vi "loadCTTAT.vi"() -> ()   [LabVIEW 2012]
uses:
  <vilib>/addons/database/Connection.llb/DB Tools Open Connec (Path).vi
  <vilib>/addons/database/Connection.llb/Conn Execute.vi
  <vilib>/addons/database/Recordset.llb/Rec Destroy - Connection.vi
  <vilib>/addons/database/Recordset.llb/Rec Fetch Recordset Data (R).vi
  <vilib>/addons/database/_DB Variant To Data/Database Variant To Data.xnode
  <vilib>/addons/database/NI_Database_API.lvlib
panel:
  out "date/time string":string
  out "recordset data":variant[][](array[variant])
  out "concatenated string":string
  out "error out":errorcluster
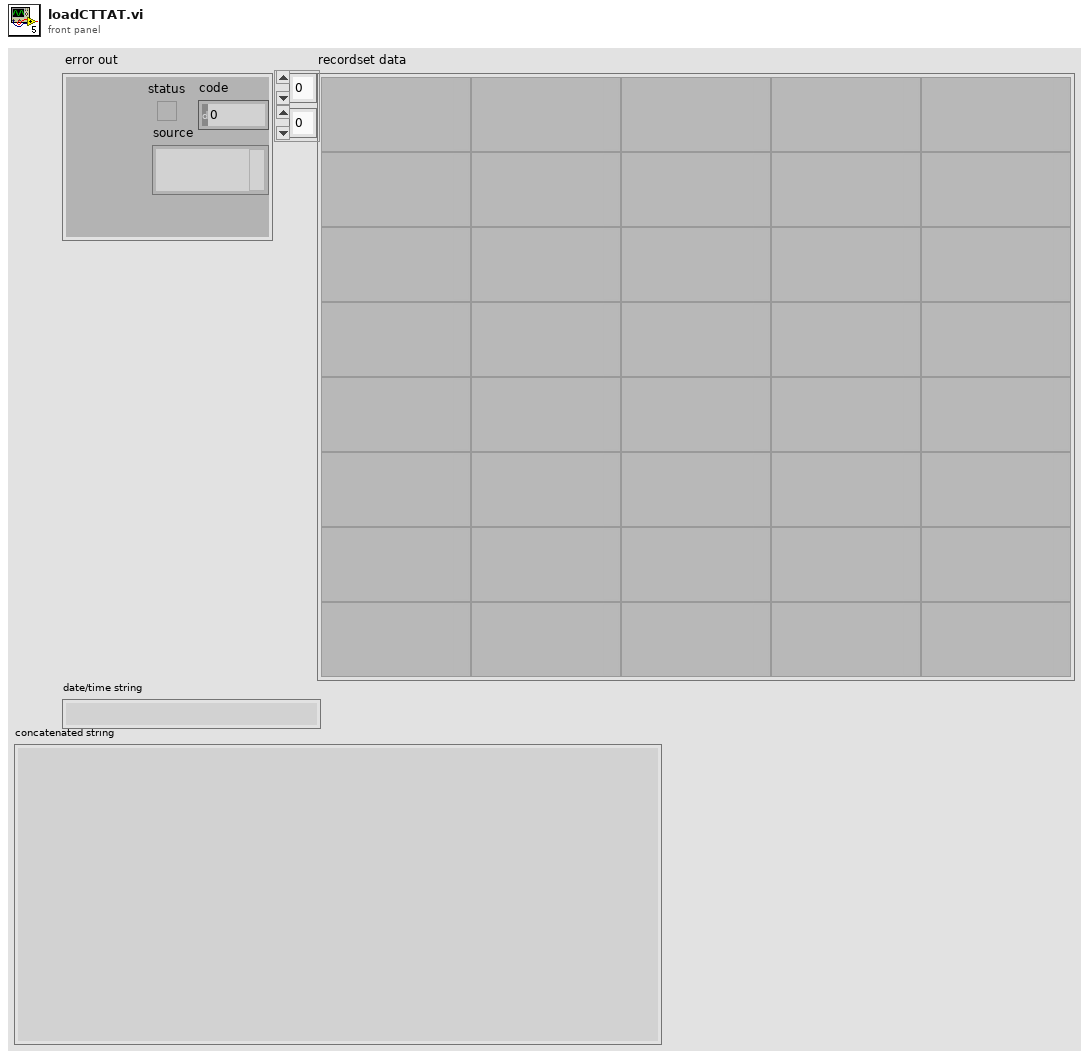
[diagram p1: front panel]
types:
  T1 = typedef "NI_Database_API.lvlib/Conn ObjectReference.ctl" = refnum<k1>
  T2 = typedef "NI_Database_API.lvlib/Rec ObjectReference.ctl" = refnum<k1>
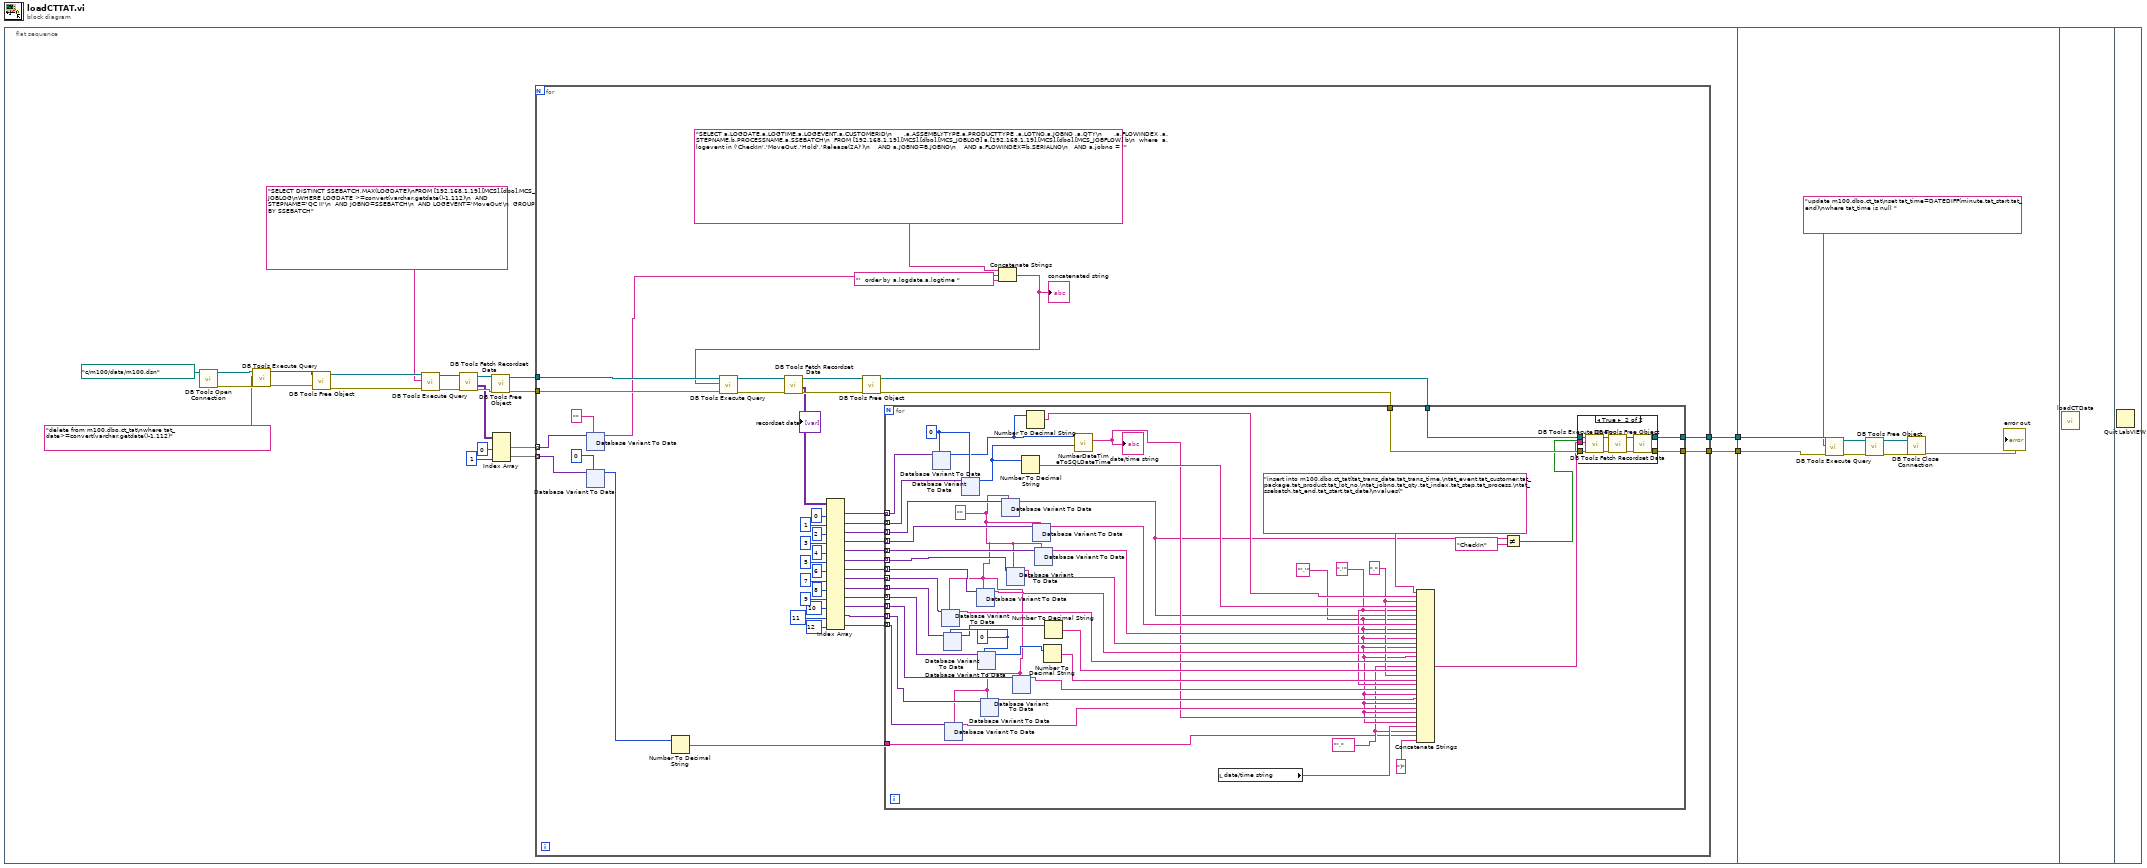
[diagram p0: block diagram]
diagram:
  n1 = flat-sequence {
    tunnel: [w4] -> w2
    tunnel: [w3] -> w1
    tunnel: w2 -> [w619]
    tunnel: w1 -> [w618]
    frame #0 {
      n2 = call-poly <vilib>:"DB Tools Open Connection.vi"("connection information"=path "c:/m100/data/m100.dsn") -> ("error out"=w9:errorcluster, "connection reference"=w12:T1)  [unwired: 7 in]
      n3 = call-poly <vilib>:"DB Tools Execute Query.vi"("error in (no error)"=w9, "SQL query"="delete from m100.dbo.ct_tat\nwhere tat_date>=convert(varchar,getdate()-1,112)", "connection reference"=w12) -> ("error out"=w8:errorcluster, "recordset reference"=w11:T2)  [unwired: 5 in]
      n4 = call-poly <vilib>:"DB Tools Free Object.vi"("error in (no error)"=w8, "recordset reference"=w11) -> ("error out"=w7:errorcluster, "connection reference"=w10:T1)  [unwired: 8 in]
      n5 = call-poly <vilib>:"DB Tools Execute Query.vi"("error in (no error)"=w7, "SQL query"="SELECT DISTINCT SSEBATCH,MAX(LOGDATE)\nFROM [192.168.1.19].[MCS].[dbo].MCS_JOBLOG\nWHERE LOGDATE >=convert(varchar,getdate()-1,112)\n  AND STEPNAME='QC II'\n  AND JOBNO=SSEBATCH\n  AND LOGEVENT='MoveOut'\n  GROUP BY SSEBATCH", "connection reference"=w10) -> ("error out"=w21:errorcluster, "recordset reference"=w23:T2)  [unwired: 5 in]
      n6 = call-poly <vilib>:"DB Tools Fetch Recordset Data.vi"("error in (no error)"=w21, "recordset reference"=w23) -> ("error out"=w20:errorcluster, "recordset data"=w19:variant[][], "recordset reference out"=w22:T2)  [unwired: 3 in]
      n7 = call-poly <vilib>:"DB Tools Free Object.vi"("error in (no error)"=w20, "recordset reference"=w22) -> ("error out"=w16:errorcluster, "connection reference"=w17:T1)  [unwired: 8 in]
      n8 = Index Array(array=w19, index (col) #1=0 ("disabled index (col)"), index (col) #2=1 ("index (col)")) -> (element #1=w15:variant[], element #2=w13:variant[])  [unwired: 2 in]
      n9 = for {
        tunnel: [w38] -> w4
        tunnel: [w37] -> w3
        tunnel: w17 -> [w36]
        tunnel: w16 -> [w35]
        tunnel: w15 -> [w34] mode=indexing
        tunnel: w13 -> [w28] mode=indexing
        n10 = xnode "Database Variant To Data"("database variant"=w34, "type"="") -> ("data"=w31:string)  [unwired: 1 in, 1 out]
        n11 = xnode "Database Variant To Data"("database variant"=w28, "type"=0) -> ("data"=w25:i32)  [unwired: 1 in, 1 out]
        n12 = Number To Decimal String(number=w25) -> (decimal integer string=w26:string)  [unwired: 1 in]
        n13 = Concatenate Strings("SELECT a.LOGDATE,a.LOGTIME,a.LOGEVENT,a.CUSTOMERID\n      ,a.ASSEMBLYTYPE,a.PRODUCTTYPE ,a.LOTNO,a.JOBNO ,a.QTY\n      ,a.FLOWINDEX ,a.STEPNAME,b.PROCESSNAME,a.SSEBATCH\n  FROM [192.168.1.19].[MCS].[dbo].[MCS_JOBLOG] a,[192.168.1.19].[MCS].[dbo].[MCS_JOBFLOW] b\n  where  a.logevent in ('CheckIn','MoveOut','Hold','Release(2A)')\n    AND a.JOBNO=B.JOBNO\n    AND a.FLOWINDEX=b.SERIALNO\n   AND a.jobno = '" ("SQL query"), w31, "'  order by a.logdate,a.logtime " ("string")) -> (w29:string)
        "concatenated string" <- w29
        n14 = call-poly <vilib>:"DB Tools Execute Query.vi"("error in (no error)"=w35, "SQL query"=w29, "connection reference"=w36) -> ("error out"=w69:errorcluster, "recordset reference"=w71:T2)  [unwired: 5 in]
        n15 = call-poly <vilib>:"DB Tools Fetch Recordset Data.vi"("error in (no error)"=w69, "recordset reference"=w71) -> ("error out"=w68:errorcluster, "recordset data"=w67:variant[][], "recordset reference out"=w70:T2)  [unwired: 3 in]
        "recordset data" <- w67
        n16 = Index Array(array=w67, index (col) #1=0 ("disabled index (col)"), index (col) #2=1 ("index (col)"), index (col) #3=2 ("index (col)"), index (col) #4=3 ("index (col)"), index (col) #5=4 ("index (col)"), index (col) #6=5 ("index (col)"), index (col) #7=6 ("index (col)"), index (col) #8=7 ("index (col)"), index (col) #9=8 ("index (col)"), index (col) #10=9 ("index (col)"), index (col) #11=10 ("index (col)"), index (col) #12=11 ("index (col)"), index (col) #13=12 ("index (col)")) -> (element #1=w55:variant[], element #2=w54:variant[], element #3=w53:variant[], element #4=w52:variant[], element #5=w51:variant[], element #6=w50:variant[], element #7=w49:variant[], element #8=w48:variant[], element #9=w47:variant[], element #10=w46:variant[], element #11=w45:variant[], element #12=w42:variant[], element #13=w41:variant[])  [unwired: 13 in]
        n17 = call-poly <vilib>:"DB Tools Free Object.vi"("error in (no error)"=w68, "recordset reference"=w70) -> ("error out"=w39:errorcluster, "connection reference"=w40:T1)  [unwired: 8 in]
        n18 = for {
          tunnel: w55 -> [w184] mode=indexing
          tunnel: w54 -> [w183] mode=indexing
          tunnel: w53 -> [w182] mode=indexing
          tunnel: w52 -> [w181] mode=indexing
          tunnel: w51 -> [w180] mode=indexing
          tunnel: w50 -> [w179] mode=indexing
          tunnel: w49 -> [w178] mode=indexing
          tunnel: w48 -> [w177] mode=indexing
          tunnel: w47 -> [w176] mode=indexing
          tunnel: w46 -> [w175] mode=indexing
          tunnel: w45 -> [w174] mode=indexing
          tunnel: w42 -> [w156] mode=indexing
          tunnel: w41 -> [w155] mode=indexing
          tunnel: w40 -> [w148]
          tunnel: w39 -> [w147]
          tunnel: [w146] -> w38
          tunnel: [w145] -> w37
          tunnel: w26 -> [w137]
          w138 = "'," ("string")
          w140 = "','" ("string")
          w150 = ",'" ("string")
          w159 = "," ("string")
          w172 = 0
          w154 = ""
          w173 = 0
          n19 = xnode "Database Variant To Data"("database variant"=w184, "type"=w173) -> ("data"=w171:i32)  [unwired: 1 in, 1 out]
          n20 = xnode "Database Variant To Data"("database variant"=w177, "type"=w154) -> ("data"=w162:string)  [unwired: 1 in, 1 out]
          n21 = xnode "Database Variant To Data"("database variant"=w176, "type"=w172) -> ("data"=w161:i32)  [unwired: 1 in, 1 out]
          n22 = xnode "Database Variant To Data"("database variant"=w155, "type"=w154) -> ("data"=w151:string)  [unwired: 1 in, 1 out]
          n23 = xnode "Database Variant To Data"("database variant"=w183, "type"=w173) -> ("data"=w170:i32)  [unwired: 1 in, 1 out]
          n24 = xnode "Database Variant To Data"("database variant"=w178, "type"=w154) -> ("data"=w163:string)  [unwired: 1 in, 1 out]
          n25 = xnode "Database Variant To Data"("database variant"=w175, "type"=w172) -> ("data"=w158:i32)  [unwired: 1 in, 1 out]
          n26 = xnode "Database Variant To Data"("database variant"=w156, "type"=w154) -> ("data"=w152:string)  [unwired: 1 in, 1 out]
          n27 = xnode "Database Variant To Data"("database variant"=w182, "type"=w154) -> ("data"=w143:string)  [unwired: 1 in, 1 out]
          n28 = xnode "Database Variant To Data"("database variant"=w179, "type"=w154) -> ("data"=w164:string)  [unwired: 1 in, 1 out]
          n29 = xnode "Database Variant To Data"("database variant"=w174, "type"=w154) -> ("data"=w153:string)  [unwired: 1 in, 1 out]
          n30 = Number To Decimal String(number=w170) -> (decimal integer string=w167:string)  [unwired: 1 in]
          n31 = Number To Decimal String(number=w171) -> (decimal integer string=w168:string)  [unwired: 1 in]
          n32 = xnode "Database Variant To Data"("database variant"=w181, "type"=w154) -> ("data"=w166:string)  [unwired: 1 in, 1 out]
          n33 = xnode "Database Variant To Data"("database variant"=w180, "type"=w154) -> ("data"=w165:string)  [unwired: 1 in, 1 out]
          n34 = Number To Decimal String(number=w158) -> (decimal integer string=w157:string)  [unwired: 1 in]
          n35 = Number To Decimal String(number=w161) -> (decimal integer string=w160:string)  [unwired: 1 in]
          n36 = call "NumberDateTimeToSQLDateTime.vi"("StartTime"=w170, "StartDate"=w171) -> ("date/time string"=w149:string)  [unwired: 9 in]
          "date/time string" <- w149
          n37 = local read "date/time string"() -> (w139:string)
          n38 = Concatenate Strings("insert into m100.dbo.ct_tat(tat_trans_date,tat_trans_time,\ntat_event,tat_customer,tat_package,tat_product,tat_lot_no,\ntat_jobno,tat_qty,tat_index,tat_step,tat_process,\ntat_ssebatch,tat_end,tat_start,tat_date)\nvalues(", w168, w159, w167, w150, w143, w140, w166, w140, w165, w140, w164, w140, w163, w140, w162, w138, w160, w159, w157, w150, w153, w140, w152, w140, w151, w140, w149, w140, w139, w138, w137, ")" ("string")) -> (w144:string)
          n39 = Not Equal?(x=w143, y="CheckIn") -> (x != y?=w141:bool)
          n40 = case shown="True" w141 {
            tunnel: w148 -> [w186 w193]
            tunnel: w147 -> [w185 w192]
            tunnel: [w186 w189] -> w146
            tunnel: [w185 w188] -> w145
            tunnel: w144 -> [_ w187]
            frame False {
            }
            frame True {
              n41 = call-poly <vilib>:"DB Tools Execute Query.vi"("error in (no error)"=w192, "SQL query"=w187, "connection reference"=w193) -> ("error out"=w191:errorcluster, "recordset reference"=w195:T2)  [unwired: 5 in]
              n42 = call-poly <vilib>:"DB Tools Fetch Recordset Data.vi"("error in (no error)"=w191, "recordset reference"=w195) -> ("error out"=w190:errorcluster, "recordset reference out"=w194:T2)  [unwired: 3 in, 1 out]
              n43 = call-poly <vilib>:"DB Tools Free Object.vi"("error in (no error)"=w190, "recordset reference"=w194) -> ("error out"=w188:errorcluster, "connection reference"=w189:T1)  [unwired: 8 in]
            }
          }
        }
      }
    }
    frame #1 {
      n44 = call-poly <vilib>:"DB Tools Execute Query.vi"("error in (no error)"=w618, "SQL query"="update m100.dbo.ct_tat\nset tat_time=DATEDIFF(minute,tat_start,tat_end)\nwhere tat_time is null ", "connection reference"=w619) -> ("error out"=w616:errorcluster, "recordset reference"=w617:T2)  [unwired: 5 in]
      n45 = call-poly <vilib>:"DB Tools Free Object.vi"("error in (no error)"=w616, "recordset reference"=w617) -> ("error out"=w612:errorcluster, "connection reference"=w613:T1)  [unwired: 8 in]
      n46 = call <vilib>:"DB Tools Close Connection.vi"("error in (no error)"=w612, "connection reference"=w613) -> ("error out"=→"error out":errorcluster)  [unwired: 5 in]
    }
    frame #2 {
      n47 = call "loadCTData.vi"() -> ()  [unwired: 12 in]
    }
    frame #3 {
      n48 = Quit LabVIEW() -> ()  [unwired: 1 in]
    }
  }
